vi "Valve_EPICS_Dev4_APX_NEXT.vi"() -> ()   [LabVIEW 2015]
uses:
  <vilib>/Platform/TimedLoop/XDataNode/timing_clust.ctl
  <vilib>/Platform/TimedLoop/XDataNode/nitl_modes.ctl
  <vilib>/Platform/TimedLoop/XDataNode/wakeup.ctl
  <userlib>/caLab/Private/Get_PV-1D.vi
  <userlib>/caLab/Private/Put_DBL-1D_PV-1D.vi
  <vilib>/platform/TimedLoop/XDataNode/XDataNode.xnode
  <vilib>/Platform/TimedLoop/XDataNode/XDNodeRunTimeDep.lvlib
panel:
  out "V7_CLOSE_REQ":bool
  out "V6_CLOSE_REQ":bool
  out "V5_CLOSE_REQ":bool
  out "V4_CLOSE_REQ":bool
  out "V3_CLOSE_REQ":bool
  out "V2_CLOSE_REQ":bool
  out "V1_CLOSE_REQ":bool
  out "V0_CLOSE_REQ":bool
  out "V7_OPEN_REQ":bool
  out "V6_OPEN_REQ":bool
  out "V5_OPEN_REQ":bool
  out "V4_OPEN_REQ":bool
  out "V3_OPEN_REQ":bool
  out "V2_OPEN_REQ":bool
  out "V1_OPEN_REQ":bool
  out "V0_OPEN_REQ":bool
  out "V7_OPEN_ENB":bool
  out "V6_OPEN_ENB":bool
  out "V5_OPEN_ENB":bool
  out "V4_OPEN_ENB":bool
  out "V3_OPEN_ENB":bool
  out "V2_OPEN_ENB":bool
  out "V1_OPEN_ENB":bool
  out "V0_OPEN_ENB":bool
  out "Boolean array":bool[](array[boolean])
  out "V7_OPEN_ACT":bool
  out "V6_OPEN_ACT":bool
  out "V5_OPEN_ACT":bool
  out "V4_OPEN_ACT":bool
  out "V3_OPEN_ACT":bool
  out "V2_OPEN_ACT":bool
  out "V1_OPEN_ACT":bool
  out "V0_OPEN_ACT":bool
  out "initialized array":i16[](array[numeric])
  in  "stop":bool
  out "sum":i16
  out "0, 1":i16[](array[numeric])
  out "SCL_data":u32[](array[numeric]) caption="SCL"
  out "SOP_data":u32[](array[numeric]) caption="SOP"
  out "SCL7":bool
  out "SCL6":bool
  out "SCL5":bool
  out "SCL4":bool
  out "SCL3":bool
  out "SCL2":bool
  out "SCL1":bool
  out "SCL0":bool
  out "SOP7":bool
  out "SOP6":bool
  out "SOP5":bool
  out "SOP4":bool
  out "SOP3":bool
  out "SOP2":bool
  out "SOP1":bool
  out "SOP0":bool
  # "Valve control DEV4"
  # "caput V0_ENABLE 1\ncaput V0_ENABLE 0"
  # "caput V0_OPEN_REQ 1\ncaput V0_OPEN_REQ 0"
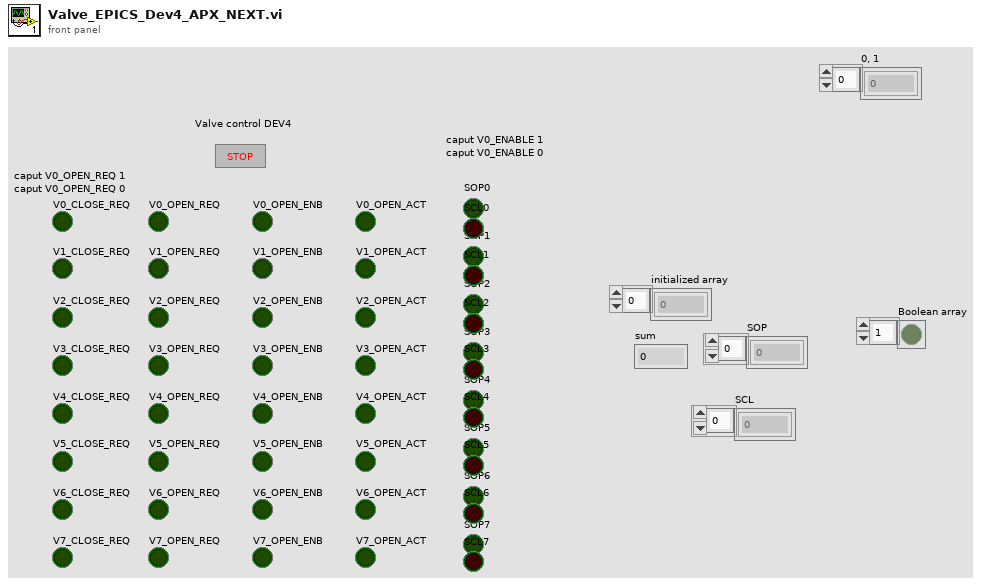
[diagram p1: front panel]
types:
  T1 = typedef "XDNodeRunTimeDep.lvlib/timing_clust.ctl" = cluster{"Expected End [f-1]":u64, "Actual End [f-1]":u64, "Finished Late? [f-1]":bool, "Expected End [i-1]":u64, "Actual End [i-1]":u64, "Finished Late? [i-1]":bool, "Expected Start [i]":u64, "Actual Start [i]":u64, "Expected Start [f]":u64, "Actual Start [f]":u64, "Source Name":string, "Structure Name":string, "Period":i64, "Deadline":i64, "Offset":i64, "Start":i64, "Priority":i32, "Timeout":i32, "Mode":T2, "Wakeup Reason":T3, "Error":errorcluster, "Source Type":string, "Secondary Source Type":string, "Global End Time":u64, "Global Start Time":u64, "Frame Duration":u64, "Iteration Duration":u64, "Assigned CPU":i32, "I/O Scan Engine Mode":u32}
  T2 = typedef "XDNodeRunTimeDep.lvlib/nitl_modes.ctl" = enum32{"No Change", "Process missed periods, maintain original phase", "Discard missed periods, maintain original phase", "Process missed periods, ignore original phase", "Discard missed periods, ignore original phase"}
  T3 = typedef "XDNodeRunTimeDep.lvlib/wakeup.ctl" = enum32{"Normal", "Aborted", "Asynchronous wakeup", "Timing source error", "Timed loop error", "Timeout"}
  T4 = typedef "NI_Matrix.lvlib/RealMatrix.ctl" = dbl[][]
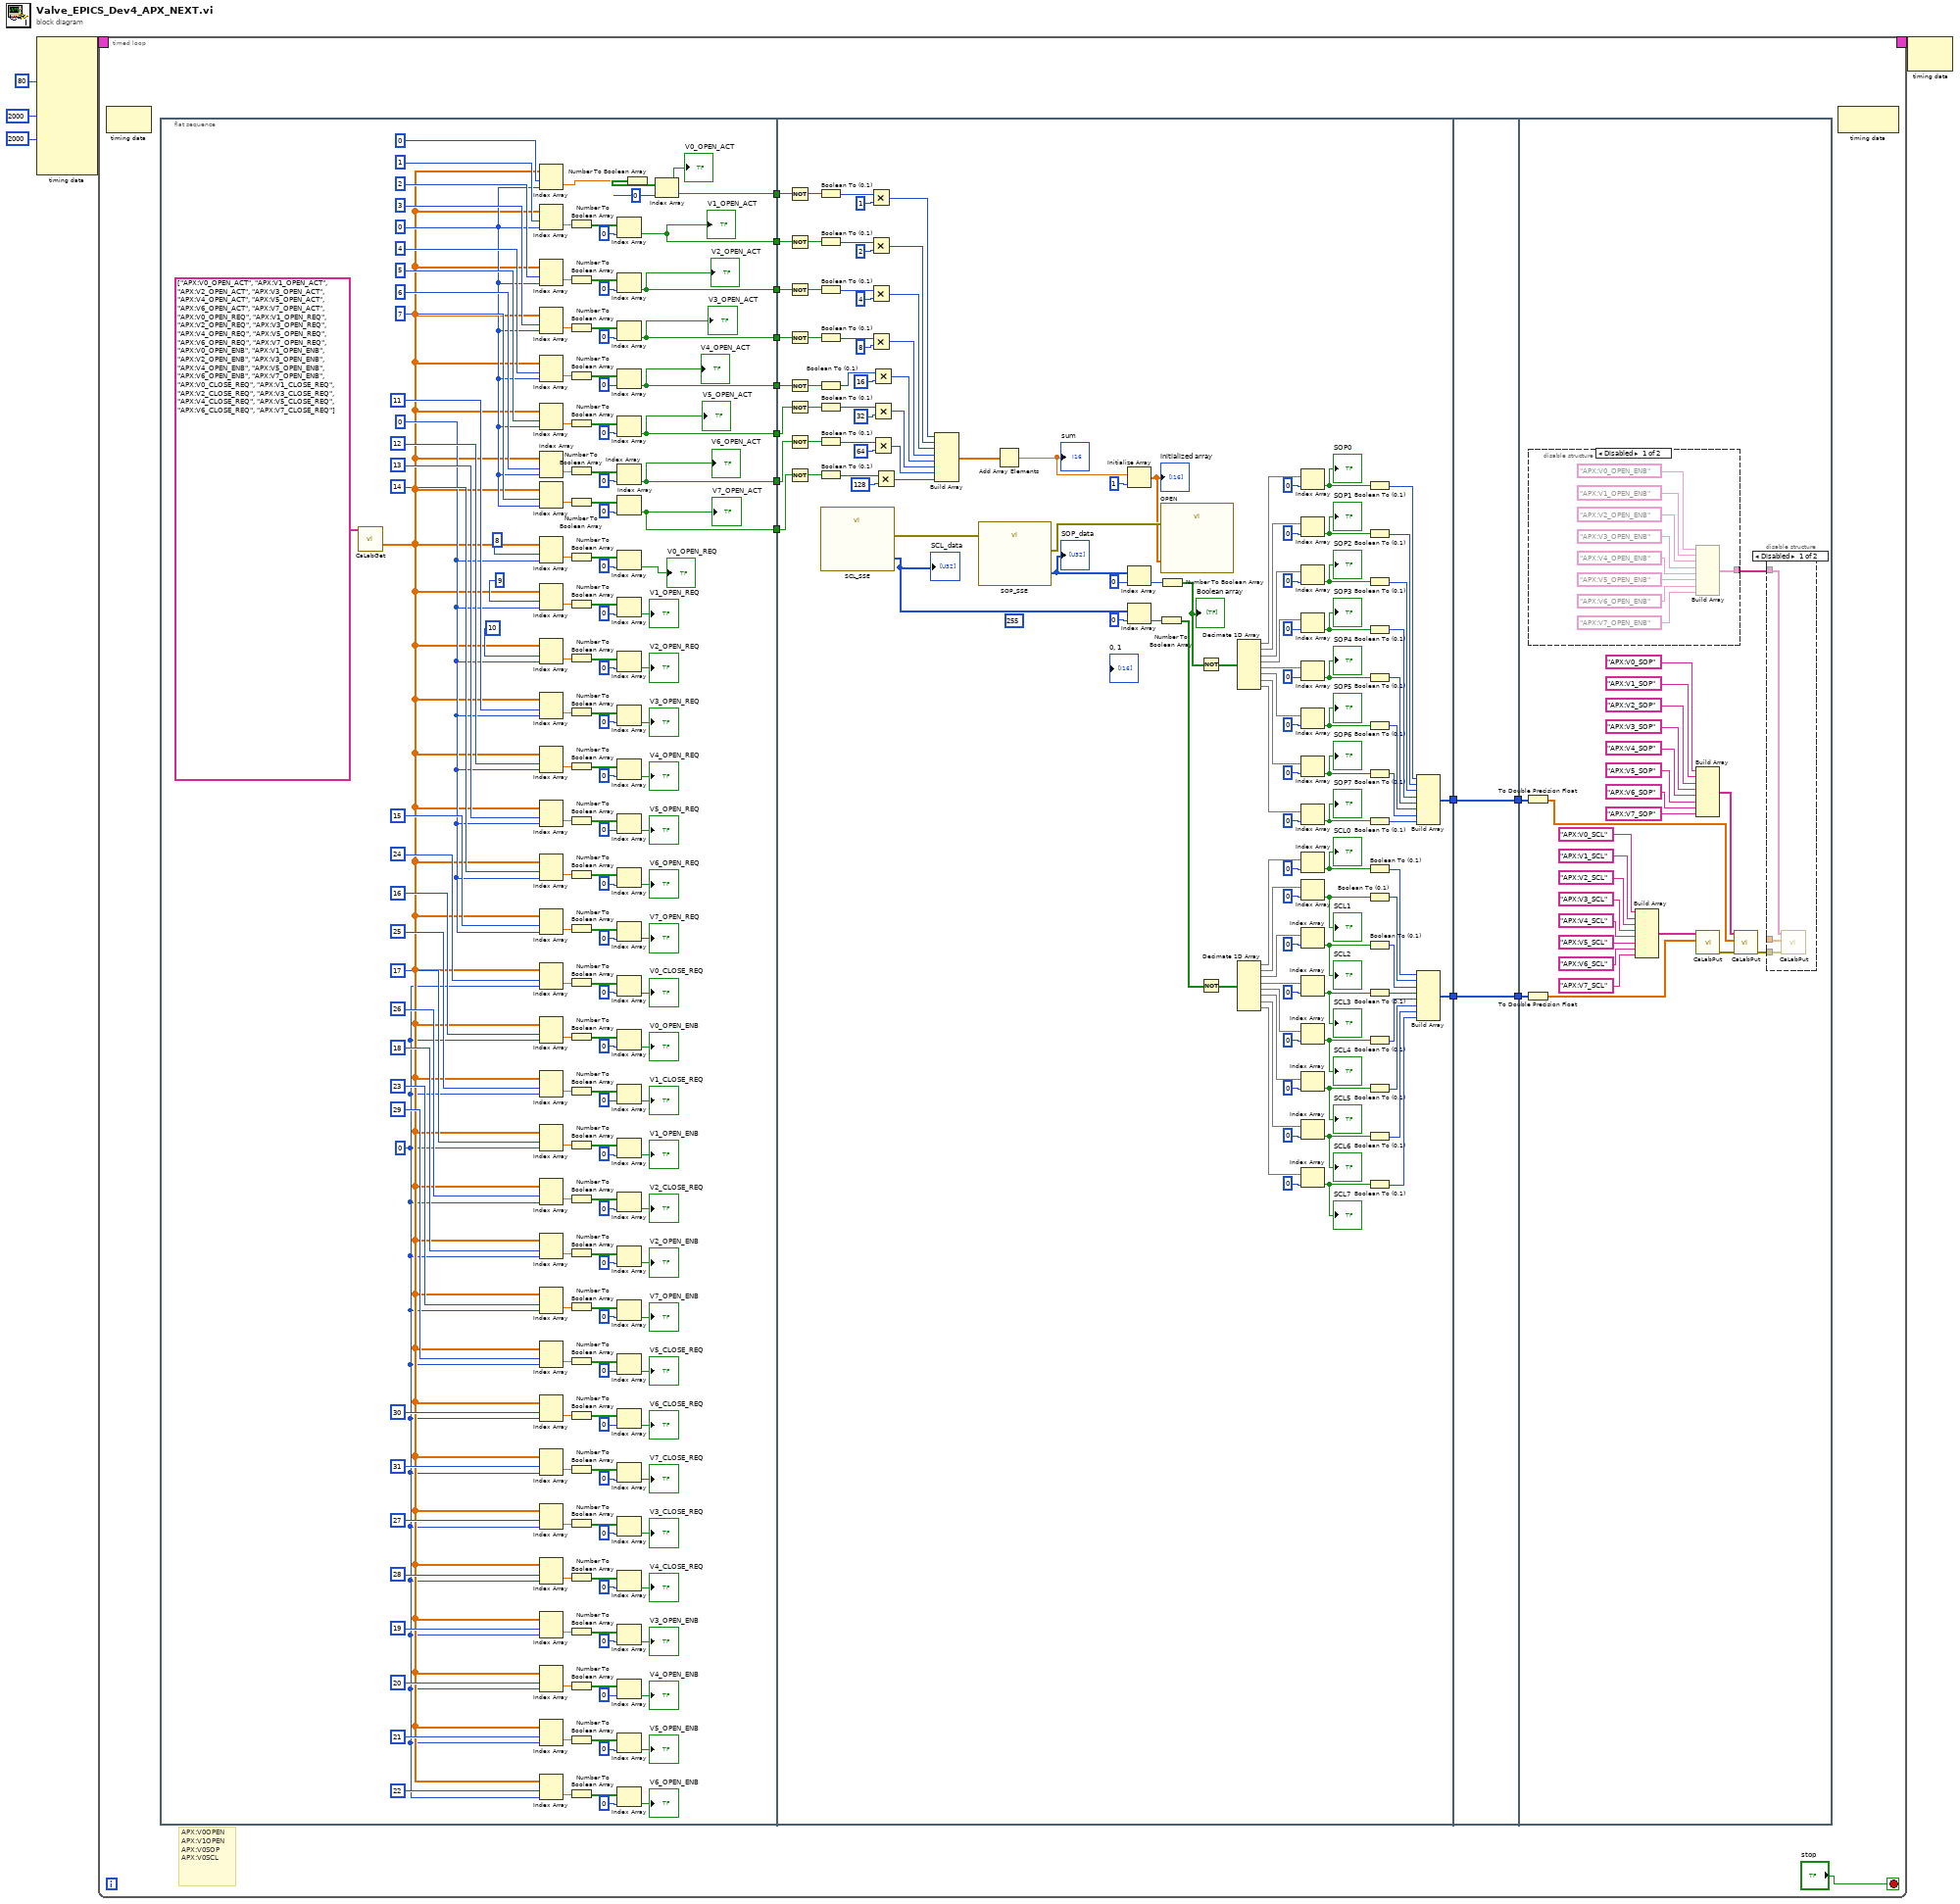
[diagram p0: block diagram]
diagram:
  n1 = node-c288(80 ("Priority"), i64 2000 ("Deadline"), 2000 ("Timeout")) -> (w5:T1)  [unwired: 7 in]
  n2 = timed-loop {
    timing: w5 -> [_]
    timing-out: [_] -> w4
    stop <- "stop" stop-if-true
    # "APX:V0OPEN\nAPX:V1OPEN\nAPX:V0SOP\nAPX:V0SCL"
    n3 = node-c288() -> ()  [unwired: 1 in, 1 out]
    n4 = flat-sequence {
      tunnel: [w68] -> w18
      tunnel: [w67] -> w17
      tunnel: [w63] -> w16
      tunnel: [w70] -> w15
      tunnel: [w69] -> w14
      tunnel: [w66] -> w13
      tunnel: [w65] -> w12
      tunnel: [w64] -> w11
      tunnel: w18 -> [w244]
      tunnel: w17 -> [w245]
      tunnel: w16 -> [w246]
      tunnel: w15 -> [w251]
      tunnel: w14 -> [w243]
      tunnel: w13 -> [w247]
      tunnel: w12 -> [w248]
      tunnel: w11 -> [w249]
      tunnel: [w195] -> w10
      tunnel: [w284] -> w7
      tunnel: w10 -> [w309]
      tunnel: [w309] -> w9
      tunnel: w7 -> [w308]
      tunnel: [w308] -> w6
      tunnel: w9 -> [w316]
      tunnel: w6 -> [w314]
      frame #0 {
        w29 = 0 ("index")
        w143 = 0 ("index")
        w176 = 0 ("index")
        n5 = call-poly "CaLabGet.vi"("PV Names"=string[] ["APX:V0_OPEN_ACT", "APX:V1_OPEN_ACT", "APX:V2_OPEN_ACT", "APX:V3_OPEN_ACT", "APX:V4_OPEN_ACT", "APX:V5_OPEN_ACT", "APX:V6_OPEN_ACT", "APX:V7_OPEN_ACT", "APX:V0_OPEN_REQ", "APX:V1_OPEN_REQ", "APX:V2_OPEN_REQ", "APX:V3_OPEN_REQ", "APX:V4_OPEN_REQ", "APX:V5_OPEN_REQ", "APX:V6_OPEN_REQ", "APX:V7_OPEN_REQ", "APX:V0_OPEN_ENB", "APX:V1_OPEN_ENB", "APX:V2_OPEN_ENB", "APX:V3_OPEN_ENB", "APX:V4_OPEN_ENB", "APX:V5_OPEN_ENB", "APX:V6_OPEN_ENB", "APX:V7_OPEN_ENB", "APX:V0_CLOSE_REQ", "APX:V1_CLOSE_REQ", "APX:V2_CLOSE_REQ", "APX:V3_CLOSE_REQ", "APX:V4_CLOSE_REQ", "APX:V5_CLOSE_REQ", "APX:V6_CLOSE_REQ", "APX:V7_CLOSE_REQ"]) -> ("Value Array (number)"=w30:dbl[][])  [unwired: 8 in, 6 out]
        n6 = Index Array(array=w30, index (row)=0 ("disabled index (row)"), index (col)=w176) -> (element=w156:dbl)
        n7 = Index Array(array=w30, index (row)=1, index (col)=w176) -> (element=w155:dbl)
        n8 = Index Array(array=w30, index (row)=2, index (col)=w176) -> (element=w159:dbl)
        n9 = Index Array(array=w30, index (row)=3 ("index"), index (col)=w176) -> (element=w158:dbl)
        n10 = Index Array(array=w30, index (row)=4, index (col)=w176) -> (element=w157:dbl)
        n11 = Index Array(array=w30, index (row)=5, index (col)=w176) -> (element=w154:dbl)
        n12 = Index Array(array=w30, index (row)=6, index (col)=w176) -> (element=w153:dbl)
        n13 = Index Array(array=w30, index (row)=7, index (col)=w176) -> (element=w152:dbl)
        n14 = Index Array(array=w30, index (row)=8 ("disabled index (row)"), index (col)=w143) -> (element=w123:dbl)
        n15 = Index Array(array=w30, index (row)=9, index (col)=w143) -> (element=w122:dbl)
        n16 = Index Array(array=w30, index (row)=10, index (col)=w143) -> (element=w126:dbl)
        n17 = Index Array(array=w30, index (row)=11 ("index"), index (col)=w143) -> (element=w125:dbl)
        n18 = Index Array(array=w30, index (row)=12, index (col)=w143) -> (element=w124:dbl)
        n19 = Index Array(array=w30, index (row)=13, index (col)=w143) -> (element=w121:dbl)
        n20 = Index Array(array=w30, index (row)=14, index (col)=w143) -> (element=w120:dbl)
        n21 = Index Array(array=w30, index (row)=15, index (col)=w143) -> (element=w119:dbl)
        n22 = Index Array(array=w30, index (row)=24, index (col)=w29) -> (element=w43:dbl)
        n23 = Index Array(array=w30, index (row)=16 ("disabled index (row)"), index (col)=w29) -> (element=w91:dbl)
        n24 = Index Array(array=w30, index (row)=25, index (col)=w29) -> (element=w42:dbl)
        n25 = Index Array(array=w30, index (row)=17, index (col)=w29) -> (element=w90:dbl)
        n26 = Index Array(array=w30, index (row)=26, index (col)=w29) -> (element=w46:dbl)
        n27 = Index Array(array=w30, index (row)=18, index (col)=w29) -> (element=w94:dbl)
        n28 = Index Array(array=w30, index (row)=23, index (col)=w29) -> (element=w87:dbl)
        n29 = Index Array(array=w30, index (row)=29, index (col)=w29) -> (element=w41:dbl)
        n30 = Index Array(array=w30, index (row)=30, index (col)=w29) -> (element=w40:dbl)
        n31 = Index Array(array=w30, index (row)=31, index (col)=w29) -> (element=w39:dbl)
        n32 = Index Array(array=w30, index (row)=27, index (col)=w29) -> (element=w45:dbl)
        n33 = Index Array(array=w30, index (row)=28, index (col)=w29) -> (element=w44:dbl)
        n34 = Index Array(array=w30, index (row)=19 ("index"), index (col)=w29) -> (element=w93:dbl)
        n35 = Index Array(array=w30, index (row)=20, index (col)=w29) -> (element=w92:dbl)
        n36 = Index Array(array=w30, index (row)=21, index (col)=w29) -> (element=w89:dbl)
        n37 = Index Array(array=w30, index (row)=22, index (col)=w29) -> (element=w88:dbl)
        n38 = Number To Boolean Array(number=w155) -> (Boolean array=w167:bool[])
        n39 = Number To Boolean Array(number=w159) -> (Boolean array=w175:bool[])
        n40 = Number To Boolean Array(number=w158) -> (Boolean array=w173:bool[])
        n41 = Number To Boolean Array(number=w157) -> (Boolean array=w171:bool[])
        n42 = Number To Boolean Array(number=w154) -> (Boolean array=w165:bool[])
        n43 = Number To Boolean Array(number=w153) -> (Boolean array=w163:bool[])
        n44 = Number To Boolean Array(number=w152) -> (Boolean array=w161:bool[])
        n45 = Number To Boolean Array(number=w123) -> (Boolean array=w136:bool[])
        n46 = Number To Boolean Array(number=w122) -> (Boolean array=w134:bool[])
        n47 = Number To Boolean Array(number=w126) -> (Boolean array=w142:bool[])
        n48 = Number To Boolean Array(number=w125) -> (Boolean array=w140:bool[])
        n49 = Number To Boolean Array(number=w124) -> (Boolean array=w138:bool[])
        n50 = Number To Boolean Array(number=w121) -> (Boolean array=w132:bool[])
        n51 = Number To Boolean Array(number=w120) -> (Boolean array=w130:bool[])
        n52 = Number To Boolean Array(number=w119) -> (Boolean array=w128:bool[])
        n53 = Number To Boolean Array(number=w43) -> (Boolean array=w56:bool[])
        n54 = Number To Boolean Array(number=w91) -> (Boolean array=w104:bool[])
        n55 = Number To Boolean Array(number=w42) -> (Boolean array=w54:bool[])
        n56 = Number To Boolean Array(number=w90) -> (Boolean array=w102:bool[])
        n57 = Number To Boolean Array(number=w46) -> (Boolean array=w62:bool[])
        n58 = Number To Boolean Array(number=w94) -> (Boolean array=w110:bool[])
        n59 = Number To Boolean Array(number=w87) -> (Boolean array=w96:bool[])
        n60 = Number To Boolean Array(number=w41) -> (Boolean array=w52:bool[])
        n61 = Number To Boolean Array(number=w40) -> (Boolean array=w50:bool[])
        n62 = Number To Boolean Array(number=w39) -> (Boolean array=w48:bool[])
        n63 = Number To Boolean Array(number=w45) -> (Boolean array=w60:bool[])
        n64 = Number To Boolean Array(number=w44) -> (Boolean array=w58:bool[])
        n65 = Number To Boolean Array(number=w93) -> (Boolean array=w108:bool[])
        n66 = Number To Boolean Array(number=w92) -> (Boolean array=w106:bool[])
        n67 = Number To Boolean Array(number=w89) -> (Boolean array=w100:bool[])
        n68 = Number To Boolean Array(number=w88) -> (Boolean array=w98:bool[])
        n69 = Index Array(array=w167, index=0) -> (element=w69:bool)
        "V1_OPEN_ACT" <- w69
        n70 = Index Array(array=w175, index=0) -> (element=w68:bool)
        "V2_OPEN_ACT" <- w68
        n71 = Index Array(array=w173, index=0) -> (element=w67:bool)
        "V3_OPEN_ACT" <- w67
        n72 = Index Array(array=w171, index=0) -> (element=w63:bool)
        "V4_OPEN_ACT" <- w63
        n73 = Index Array(array=w165, index=0) -> (element=w66:bool)
        "V5_OPEN_ACT" <- w66
        n74 = Index Array(array=w163, index=0) -> (element=w65:bool)
        "V6_OPEN_ACT" <- w65
        n75 = Index Array(array=w161, index=0) -> (element=w64:bool)
        "V7_OPEN_ACT" <- w64
        n76 = Index Array "Index Array"(array=w136, index=0) -> (element=→"V0_OPEN_REQ":bool)
        n77 = Index Array(array=w134, index=0) -> (element=→"V1_OPEN_REQ":bool)
        n78 = Index Array(array=w142, index=0) -> (element=→"V2_OPEN_REQ":bool)
        n79 = Index Array(array=w140, index=0) -> (element=→"V3_OPEN_REQ":bool)
        n80 = Index Array(array=w138, index=0) -> (element=→"V4_OPEN_REQ":bool)
        n81 = Index Array(array=w132, index=0) -> (element=→"V5_OPEN_REQ":bool)
        n82 = Index Array(array=w130, index=0) -> (element=→"V6_OPEN_REQ":bool)
        n83 = Index Array(array=w128, index=0) -> (element=→"V7_OPEN_REQ":bool)
        n84 = Index Array(array=w56, index=0) -> (element=→"V0_CLOSE_REQ":bool)
        n85 = Index Array(array=w104, index=0) -> (element=→"V0_OPEN_ENB":bool)
        n86 = Index Array(array=w54, index=0) -> (element=→"V1_CLOSE_REQ":bool)
        n87 = Index Array(array=w102, index=0) -> (element=→"V1_OPEN_ENB":bool)
        n88 = Index Array(array=w62, index=0) -> (element=→"V2_CLOSE_REQ":bool)
        n89 = Index Array(array=w110, index=0) -> (element=→"V2_OPEN_ENB":bool)
        n90 = Index Array(array=w96, index=0) -> (element=→"V7_OPEN_ENB":bool)
        n91 = Index Array(array=w52, index=0) -> (element=→"V5_CLOSE_REQ":bool)
        n92 = Index Array(array=w50, index=0) -> (element=→"V6_CLOSE_REQ":bool)
        n93 = Index Array(array=w48, index=0) -> (element=→"V7_CLOSE_REQ":bool)
        n94 = Index Array(array=w60, index=0) -> (element=→"V3_CLOSE_REQ":bool)
        n95 = Index Array(array=w58, index=0) -> (element=→"V4_CLOSE_REQ":bool)
        n96 = Index Array(array=w108, index=0) -> (element=→"V3_OPEN_ENB":bool)
        n97 = Index Array(array=w106, index=0) -> (element=→"V4_OPEN_ENB":bool)
        n98 = Index Array(array=w100, index=0) -> (element=→"V5_OPEN_ENB":bool)
        n99 = Index Array(array=w98, index=0) -> (element=→"V6_OPEN_ENB":bool)
        n100 = Number To Boolean Array(number=w156) -> (Boolean array=w169:bool[])
        n101 = Index Array(array=w169, index=0) -> (element=w70:bool)
        "V0_OPEN_ACT" <- w70
      }
      frame #1 {
        (unwired) u32 255 ("y")
        n102 = Not(x=w251) -> (.not. x?=w250:bool)
        n103 = Not(x=w243) -> (.not. x?=w275:bool)
        n104 = Not(x=w244) -> (.not. x?=w274:bool)
        n105 = Not(x=w245) -> (.not. x?=w273:bool)
        n106 = Not(x=w246) -> (.not. x?=w272:bool)
        n107 = Not(x=w247) -> (.not. x?=w271:bool)
        n108 = Not(x=w248) -> (.not. x?=w270:bool)
        n109 = Not(x=w249) -> (.not. x?=w269:bool)
        n110 = Boolean To (0,1)(Boolean=w250) -> (0, 1=w283:i16)
        n111 = Boolean To (0,1)(Boolean=w275) -> (0, 1=w282:i16)
        n112 = Boolean To (0,1)(Boolean=w274) -> (0, 1=w281:i16)
        n113 = Boolean To (0,1)(Boolean=w273) -> (0, 1=w280:i16)
        n114 = Boolean To (0,1)(Boolean=w272) -> (0, 1=w279:i16)
        n115 = Boolean To (0,1)(Boolean=w271) -> (0, 1=w278:i16)
        n116 = Boolean To (0,1)(Boolean=w270) -> (0, 1=w277:i16)
        n117 = Boolean To (0,1)(Boolean=w269) -> (0, 1=w276:i16)
        n118 = call "SCL_SSE"() -> ("data"=w223:u32[], "error out"=w298:errorcluster)  [unwired: 17 in, 1 out]
        "SCL_data" <- w223
        n119 = Multiply(x=w283, y=i16 1) -> (x*y=w260:i16)
        n120 = Multiply(x=w282, y=i16 2) -> (x*y=w259:i16)
        n121 = Multiply(x=w281, y=i16 4) -> (x*y=w258:i16)
        n122 = Multiply(x=w280, y=i16 8) -> (x*y=w257:i16)
        n123 = Multiply(x=w279, y=i16 16) -> (x*y=w256:i16)
        n124 = Multiply(x=w278, y=i16 32) -> (x*y=w255:i16)
        n125 = Multiply(x=w277, y=i16 64) -> (x*y=w254:i16)
        n126 = Multiply(x=w276, y=i16 128) -> (x*y=w253:i16)
        n127 = Build Array(w260, w259, w258, w257, w256, w255, w254, w253) -> (w252:T4)
        n128 = call "SOP_SSE"("error in"=w298) -> ("data"=w222:u32[], "error out"=w297:errorcluster)  [unwired: 16 in, 1 out]
        "SOP_data" <- w222
        n129 = Add Array Elements(numeric array=w252) -> (sum=w295:dbl)
        "sum" <- w295
        n130 = Initialize Array(w295, 1 ("dimension size")) -> (w294:dbl[])
        "initialized array" <- w294
        n131 = Index Array(array=w222, index=0) -> (element=w242:u32)
        n132 = Index Array(array=w223, index=0) -> (element=w241:u32)
        n133 = Number To Boolean Array(number=w241) -> (Boolean array=w232:bool[])
        n134 = call "OPEN"("data"=w294, "error in"=w297) -> ()  [unwired: 16 in, 2 out]
        n135 = Number To Boolean Array(number=w242) -> (Boolean array=w221:bool[])
        "Boolean array" <- w221
        n136 = Not(x=w221) -> (.not. x?=w220:bool[])
        n137 = Not(x=w232) -> (.not. x?=w219:bool[])
        n138 = Decimate 1D Array(w220) -> (w240:bool[], w239:bool[], w238:bool[], w237:bool[], w236:bool[], w235:bool[], w234:bool[], w233:bool[])
        n139 = Decimate 1D Array(w219) -> (w231:bool[], w230:bool[], w229:bool[], w228:bool[], w227:bool[], w226:bool[], w225:bool[], w224:bool[])
        n140 = Index Array(array=w240, index=0) -> (element=w203:bool)
        "SOP0" <- w203
        n141 = Index Array(array=w239, index=0) -> (element=w218:bool)
        "SOP1" <- w218
        n142 = Index Array(array=w238, index=0) -> (element=w210:bool)
        "SOP2" <- w210
        n143 = Index Array(array=w237, index=0) -> (element=w209:bool)
        "SOP3" <- w209
        n144 = Index Array(array=w236, index=0) -> (element=w208:bool)
        "SOP4" <- w208
        n145 = Index Array(array=w235, index=0) -> (element=w207:bool)
        "SOP5" <- w207
        n146 = Index Array(array=w234, index=0) -> (element=w206:bool)
        "SOP6" <- w206
        n147 = Index Array(array=w233, index=0) -> (element=w205:bool)
        "SOP7" <- w205
        n148 = Index Array(array=w231, index=0) -> (element=w193:bool)
        "SCL0" <- w193
        n149 = Index Array(array=w230, index=0) -> (element=w192:bool)
        "SCL1" <- w192
        n150 = Index Array(array=w229, index=0) -> (element=w191:bool)
        "SCL2" <- w191
        n151 = Index Array(array=w228, index=0) -> (element=w190:bool)
        "SCL3" <- w190
        n152 = Index Array(array=w227, index=0) -> (element=w189:bool)
        "SCL4" <- w189
        n153 = Index Array(array=w226, index=0) -> (element=w188:bool)
        "SCL5" <- w188
        n154 = Index Array(array=w225, index=0) -> (element=w187:bool)
        "SCL6" <- w187
        n155 = Index Array(array=w224, index=0) -> (element=w186:bool)
        "SCL7" <- w186
        n156 = Boolean To (0,1)(Boolean=w203) -> (0, 1=w204:i16)
        n157 = Boolean To (0,1)(Boolean=w218) -> (0, 1=w217:i16)
        n158 = Boolean To (0,1)(Boolean=w210) -> (0, 1=w216:i16)
        n159 = Boolean To (0,1)(Boolean=w209) -> (0, 1=w215:i16)
        n160 = Boolean To (0,1)(Boolean=w208) -> (0, 1=w214:i16)
        n161 = Boolean To (0,1)(Boolean=w207) -> (0, 1=w213:i16)
        n162 = Boolean To (0,1)(Boolean=w206) -> (0, 1=w212:i16)
        n163 = Boolean To (0,1)(Boolean=w205) -> (0, 1=w211:i16)
        n164 = Boolean To (0,1)(Boolean=w193) -> (0, 1=w196:i16)
        n165 = Boolean To (0,1)(Boolean=w192) -> (0, 1=w202:i16)
        n166 = Boolean To (0,1)(Boolean=w191) -> (0, 1=w201:i16)
        n167 = Boolean To (0,1)(Boolean=w190) -> (0, 1=w200:i16)
        n168 = Boolean To (0,1)(Boolean=w189) -> (0, 1=w199:i16)
        n169 = Boolean To (0,1)(Boolean=w188) -> (0, 1=w198:i16)
        n170 = Boolean To (0,1)(Boolean=w187) -> (0, 1=w197:i16)
        n171 = Boolean To (0,1)(Boolean=w186) -> (0, 1=w194:i16)
        n172 = Build Array(w204, w217, w216, w215, w214, w213, w212, w211) -> (w284:i16[])
        n173 = Build Array(w196, w202, w201, w200, w199, w198, w197, w194) -> (w195:i16[])
      }
      frame #2 {
      }
      frame #3 {
        n174 = To Double Precision Float(number=w314) -> (double precision float=w317:dbl[])
        n175 = To Double Precision Float(number=w316) -> (double precision float=w315:dbl[])
        n176 = disable-structure shown="Disabled" {
          disable-tunnel: [w338 _] -> w312
          frame Disabled {
            n177 = Build Array("APX:V0_OPEN_ENB", "APX:V1_OPEN_ENB", "APX:V2_OPEN_ENB", "APX:V3_OPEN_ENB", "APX:V4_OPEN_ENB", "APX:V5_OPEN_ENB", "APX:V6_OPEN_ENB", "APX:V7_OPEN_ENB") -> (w338:string[])
          }
          frame Enabled {
          }
        }
        n178 = Build Array("APX:V0_SCL", "APX:V1_SCL", "APX:V2_SCL", "APX:V3_SCL", "APX:V4_SCL", "APX:V5_SCL", "APX:V6_SCL", "APX:V7_SCL") -> (w318:string[])
        n179 = Build Array("APX:V0_SOP", "APX:V1_SOP", "APX:V2_SOP", "APX:V3_SOP", "APX:V4_SOP", "APX:V5_SOP", "APX:V6_SOP", "APX:V7_SOP") -> (w313:string[])
        n180 = call-poly <userlib>:"CaLabPut.vi"("Values"=w315, "PV Names"=w318) -> ("Error out"=w310:errorcluster)  [unwired: 6 in, 3 out]
        n181 = call-poly <userlib>:"CaLabPut.vi"("Error in (no error)"=w310, "Values"=w317, "PV Names"=w313) -> ("Error out"=w311:errorcluster)  [unwired: 5 in, 3 out]
        n182 = disable-structure shown="Disabled" {
          disable-tunnel: _ -> [w337 _]
          disable-tunnel: w312 -> [w336 _]
          disable-tunnel: w311 -> [w335 _]
          frame Disabled {
            n183 = call-poly <userlib>:"CaLabPut.vi"("Error in (no error)"=w335, "Values"=w337, "PV Names"=w336) -> ()  [unwired: 5 in, 4 out]
          }
          frame Enabled {
          }
        }
      }
    }
    n184 = node-c288() -> ()  [unwired: 1 in, 1 out]
  }
  n185 = node-c288(w4) -> ()  [unwired: 1 out]
